vi "GenBlock.vi"(1 "编号":i8 min=-1 max=14, 2 "颜色":u32) -> (0 "输出":cluster{"编号":i8, "方块":u32[][]})   [LabVIEW 2016]
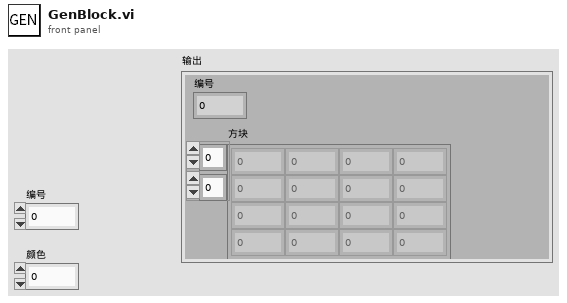
[diagram p1: front panel]
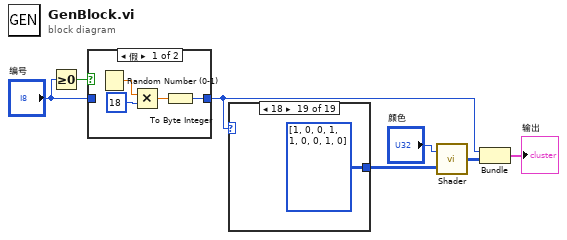
[diagram p0: block diagram]
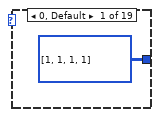
[diagram p2: hidden frame]
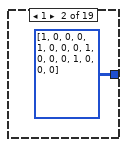
[diagram p3: hidden frame]
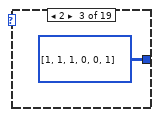
[diagram p4: hidden frame]
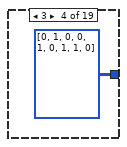
[diagram p5: hidden frame]
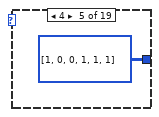
[diagram p6: hidden frame]
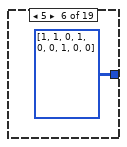
[diagram p7: hidden frame]
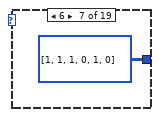
[diagram p8: hidden frame]
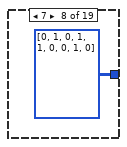
[diagram p9: hidden frame]
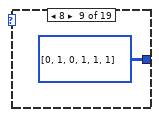
[diagram p10: hidden frame]
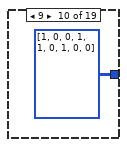
[diagram p11: hidden frame]
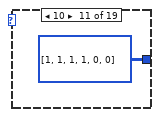
[diagram p12: hidden frame]
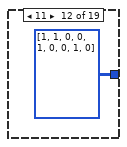
[diagram p13: hidden frame]
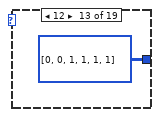
[diagram p14: hidden frame]
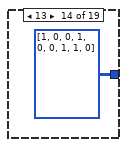
[diagram p15: hidden frame]
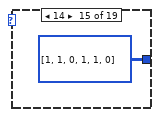
[diagram p16: hidden frame]
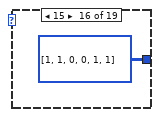
[diagram p17: hidden frame]
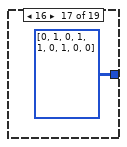
[diagram p18: hidden frame]
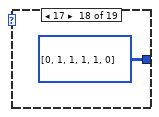
[diagram p19: hidden frame]
diagram:
  n1 = Greater Or Equal To 0?(x="编号") -> (x >= 0?=w6:bool)
  n2 = case shown="假" w6 {
    tunnel: [w8 w12] -> w4
    tunnel: "编号" -> [_ w12]
    frame False {
      n3 = Random Number (0-1)() -> (number: 0 to 1=w11:dbl)
      n4 = Multiply(x=w11, y=18) -> (x*y=w9:dbl)
      n5 = To Byte Integer(number=w9) -> (8bit integer=w8:i8)
    }
    frame True {
    }
  }
  n6 = case shown="18" w4 {
    tunnel: [i32[][] [[1, 1, 1, 1]] i32[][] [[1, 0, 0, 0], [1, 0, 0, 0], [1, 0, 0, 0], [1, 0, 0, 0]] i32[][] [[1, 1, 1], [0, 0, 1]] i32[][] [[0, 1, 0], [0, 1, 0], [1, 1, 0]] i32[][] [[1, 0, 0], [1, 1, 1]] i32[][] [[1, 1, 0], [1, 0, 0], [1, 0, 0]] i32[][] [[1, 1, 1], [0, 1, 0]] i32[][] [[0, 1, 0], [1, 1, 0], [0, 1, 0]] i32[][] [[0, 1, 0], [1, 1, 1]] i32[][] [[1, 0, 0], [1, 1, 0], [1, 0, 0]] i32[][] [[1, 1, 1], [1, 0, 0]] i32[][] [[1, 1, 0], [0, 1, 0], [0, 1, 0]] i32[][] [[0, 0, 1], [1, 1, 1]] i32[][] [[1, 0, 0], [1, 0, 0], [1, 1, 0]] i32[][] [[1, 1, 0], [1, 1, 0]] i32[][] [[1, 1, 0], [0, 1, 1]] i32[][] [[0, 1, 0], [1, 1, 0], [1, 0, 0]] i32[][] [[0, 1, 1], [1, 1, 0]] u32[][] [[1, 0, 0], [1, 1, 0], [0, 1, 0]]] -> w3
    frame 0, Default {
    }
    frame 1 {
    }
    frame 2 {
    }
    frame 3 {
    }
    frame 4 {
    }
    frame 5 {
    }
    frame 6 {
    }
    frame 7 {
    }
    frame 8 {
    }
    frame 9 {
    }
    frame 10 {
    }
    frame 11 {
    }
    frame 12 {
    }
    frame 13 {
    }
    frame 14 {
    }
    frame 15 {
    }
    frame 16 {
    }
    frame 17 {
    }
    frame 18 {
    }
  }
  n7 = call "Shader.vi"("输入"=w3, "颜色"="颜色") -> ("输出"=w2:u32[][])
  n8 = Bundle("编号"=w4, "输出"=w2) -> (→"输出":cluster{"编号":i8, "输出":u32[][]})  [unwired: 1 in]
